vi "repeat cycle_linear up.vi"(8 "error in (no error)":errorcluster caption="에러 입력(에러 없음)", 10 "waveform in":waveform(dbl), 11 "Waveform Obj 입력":refnum<class "Waveform Gen.lvclass">) -> (0 "error out":errorcluster caption="에러 출력", 2 "waveform out":waveform(dbl), 3 "Waveform Obj 출력":refnum<class "Waveform Gen.lvclass">)   [LabVIEW 2020, in "Waveform Gen.lvclass"]
uses:
  Waveform Gen.lvclass
  Waveform Gen.lvclass/Waveform Gen.ctl
  Accessors/Read cycle.vi
  <vilib>/Waveform/WDTOps.llb/WDT Append Waveforms DBL.vi
  <vilib>/Waveform/WDTOps.llb/WDT Number of Waveform Samples DBL.vi
  <vilib>/Waveform/WDTOps.llb/WDT Get Waveform Subset DBL.vi
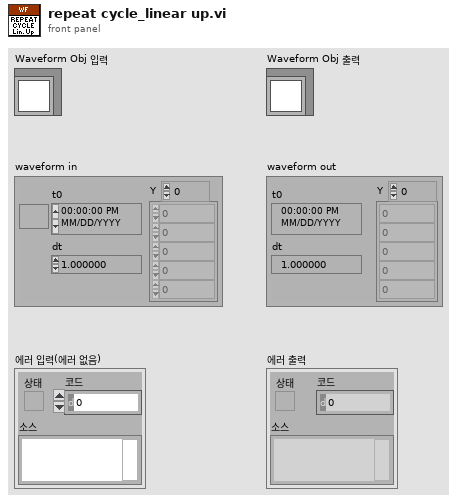
[diagram p1: front panel]
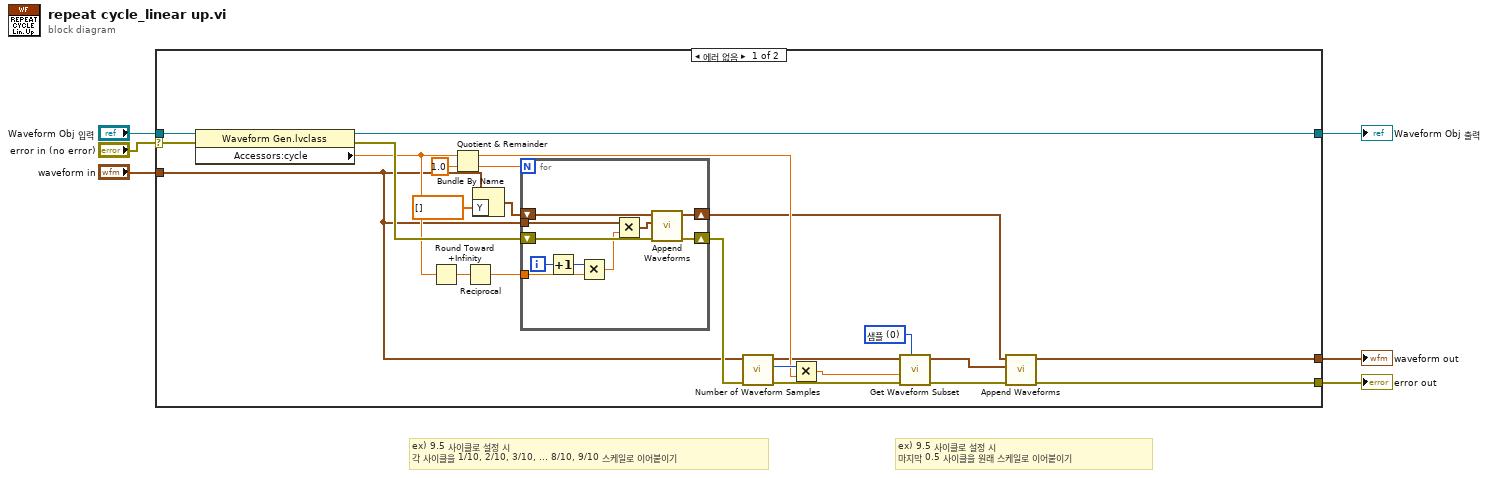
[diagram p0: block diagram]
diagram:
  # "ex) 9.5 사이클로 설정 시 \n마지막 0.5 사이클을 원래 스케일로 이어붙이기"
  # "ex) 9.5 사이클로 설정 시 \n각 사이클을 1/10, 2/10, 3/10, ... 8/10, 9/10 스케일로 이어붙이기"
  n1 = case shown="에러 없음" "error in (no error)" {
    selector: "error in (no error)" -> [w28 w42]
    tunnel: [w8 w42] -> w3
    tunnel: "Waveform Obj 입력" -> [w30 w41]
    tunnel: [w9 w41] -> w5
    tunnel: "waveform in" -> [w10 _]
    tunnel: [w7 _] -> w1
    frame No Error {
      w18 = u16 0 items=["샘플", "상대 시간"] ("start/duration format")
      n2 = property class="Waveform Gen.lvclass"(reference=w30, error in=w28) -> (reference out=w9:refnum<class "Waveform Gen.lvclass">, error out=w21:errorcluster, "Accessors:cycle"=w16:dbl)
      n3 = Round Toward +Infinity(x=w16) -> (ceil(x): smallest int >= x=w17:dbl)
      n4 = Quotient & Remainder(x=w16, y=1.0) -> (x-y*floor(x/y)=w25:dbl, floor(x/y)=w27:dbl)
      n5 = Reciprocal(x=w17) -> (1/x=w15:dbl)
      n6 = Bundle By Name(cluster=w10, "Y"=dbl[] []) -> (w12:waveform(dbl))
      n7 = for {
        N: w27 -> [_]
        shift-right: [w39] -> w13
        shift-left: w12 -> [w40]
        shift-right: [w37] -> w20
        shift-left: w21 -> [w38]
        tunnel: w10 -> [w36]
        tunnel: w15 -> [w35]
        i -> [w32]
        n8 = Increment(x=w32) -> (x+1=w31:i32)
        n9 = Multiply(x=w31, y=w35) -> (x*y=w33:dbl)
        n10 = Multiply(x=w36, y=w33) -> (x*y=w34:waveform(dbl))
        n11 = call-poly <vilib>:"Append Waveforms.vi"("error in (no error)"=w38, "waveform B"=w34, "waveform A"=w40) -> ("error out"=w37:errorcluster, "waveform out"=w39:waveform(dbl))  [unwired: 7 in]
      }
      n12 = call-poly <vilib>:"Number of Waveform Samples.vi"("error in (no error)"=w20, "waveform in"=w10) -> ("error out"=w23:errorcluster, "number of samples"=w26:i32, "waveform out"=w14:waveform(dbl))  [unwired: 7 in]
      n13 = Multiply(x=w26, y=w25) -> (x*y=w24:dbl)
      n14 = call-poly <vilib>:"Get Waveform Subset.vi"("start/duration format"=w18, "error in (no error)"=w23, "duration"=w24, "waveform in"=w14) -> ("error out"=w19:errorcluster, "waveform out"=w22:waveform(dbl))  [unwired: 2 in, 2 out]
      n15 = call-poly <vilib>:"Append Waveforms.vi"("error in (no error)"=w19, "waveform B"=w22, "waveform A"=w13) -> ("error out"=w8:errorcluster, "waveform out"=w7:waveform(dbl))  [unwired: 7 in]
    }
    frame Error {
    }
  }
  "error out" <- w3
  "Waveform Obj 출력" <- w5
  "waveform out" <- w1
